vi "Add Component Default Settings.vi"(8 "error in (no error)":errorcluster, 10 "Component":refnum<class "Component.lvclass">, 11 "framework configuration in":T1) -> (0 "error out":errorcluster, 3 "framework configuration out":T1)   [LabVIEW 2017, in "DSF Core.lvlib"]
uses:
  DSF Core.lvlib
  Typedefs/DSF Engine Framework Configuration.ctl
  Typedefs/DSF Settings Info.ctl
  Typedefs/DSF Engine Plugin Configuration.ctl
  Typedefs/DSF Engine Plugin Thread Configuration.ctl
  Typedefs/DSF Engine Transfer Group Configuration.ctl
  Typedefs/DSF Engine Transfer Configuration.ctl
  Typedefs/DSF Engine Channel Configuration.ctl
  Classes/Component/Component.lvclass
  Classes/Configuration/Base/Group/Group Configuration.lvclass
  Classes/Configuration/Configuration.lvclass
  Classes/Component Configuration/Component Configurations.lvclass
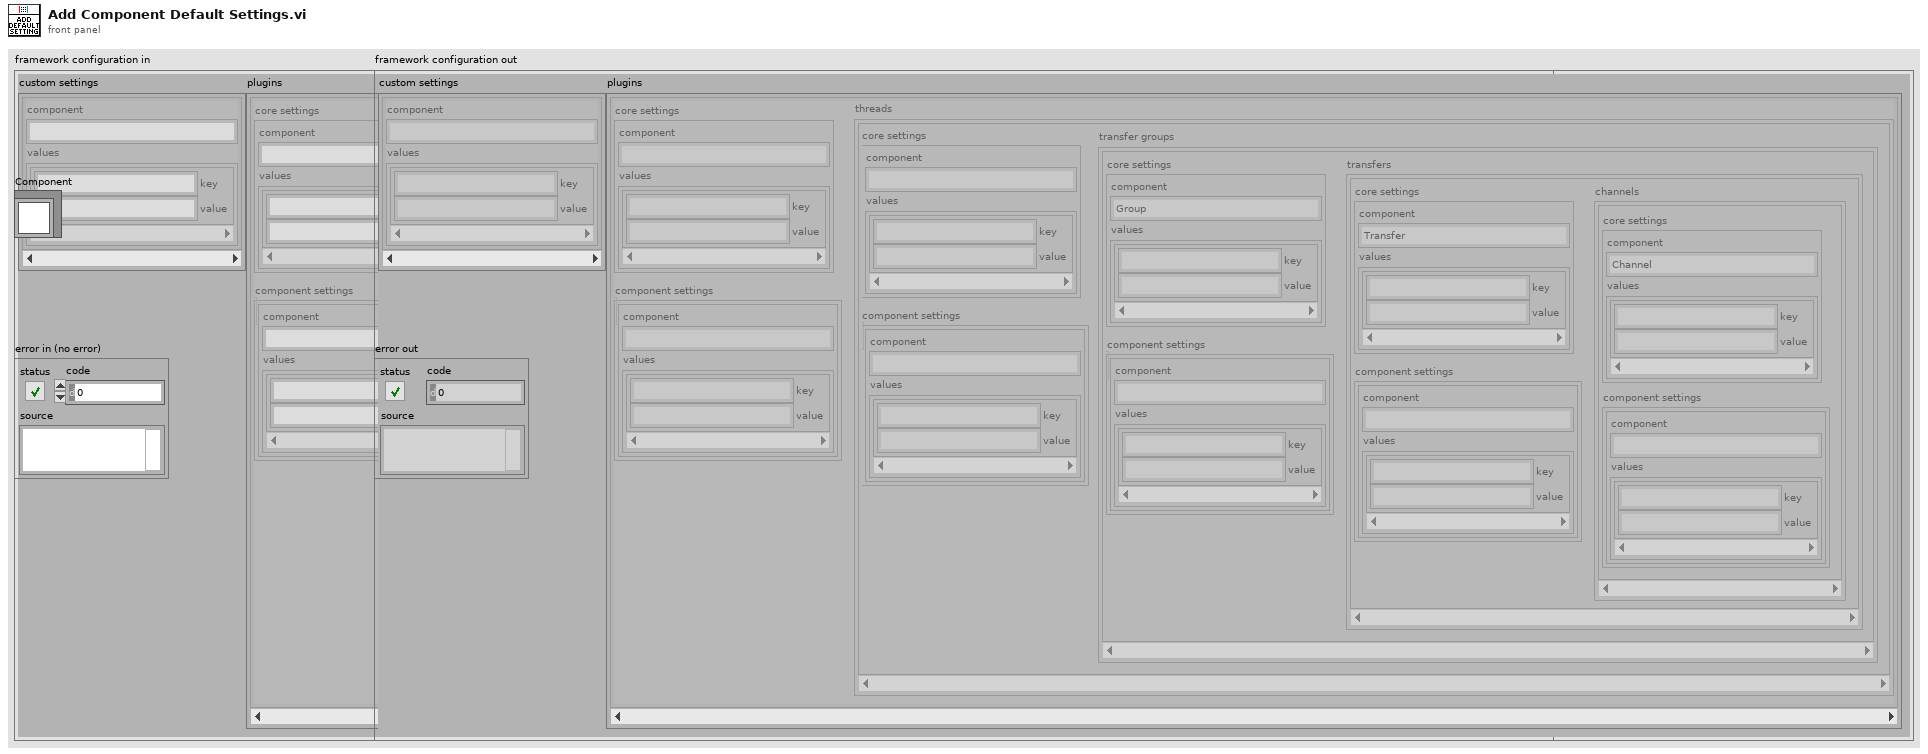
[diagram p1: front panel]
types:
  T1 = typedef "DSF Core.lvlib/DSF Engine Framework Configuration.ctl" = cluster{"custom settings":T2[], "plugins":T3[]}
  T2 = typedef "DSF Core.lvlib/DSF Settings Info.ctl" = cluster{"component":string, "values":cluster{"key":string, "value":string}[]}
  T3 = typedef "DSF Core.lvlib/DSF Engine Plugin Configuration.ctl" = cluster{"core settings":T2, "component settings":T2[], "threads":T4[]}
  T4 = typedef "DSF Core.lvlib/DSF Engine Plugin Thread Configuration.ctl" = cluster{"core settings":T2, "component settings":T2[], "transfer groups":T5[]}
  T5 = typedef "DSF Core.lvlib/DSF Engine Transfer Group Configuration.ctl" = cluster{"core settings":T2, "component settings":T2[], "transfers":T6[]}
  T6 = typedef "DSF Core.lvlib/DSF Engine Transfer Configuration.ctl" = cluster{"core settings":T2, "component settings":T2[], "channels":T7[]}
  T7 = typedef "DSF Core.lvlib/DSF Engine Channel Configuration.ctl" = cluster{"core settings":T2, "component settings":T2[]}
  T8 = typedef "DSF Core.lvlib/Group Configuration.lvclass/Core Group Configuration.ctl" = cluster{"name":string, "direction":T9, "cycle timing":T10, "timeout behavior":T11, "enable conversion":bool}
  T9 = typedef "DSF Core.lvlib/DSF Direction.ctl" = enum8{"Tx", "Rx"}
  T10 = typedef "DSF Core.lvlib/DSF Timing Info.ctl" = cluster{"priority":u64, "decimation":u64, "offset":u64}
  T11 = typedef "DSF Core.lvlib/DSF Timeout Behavior.ctl" = enum8{"Increment Late Count", "Throw Error"}
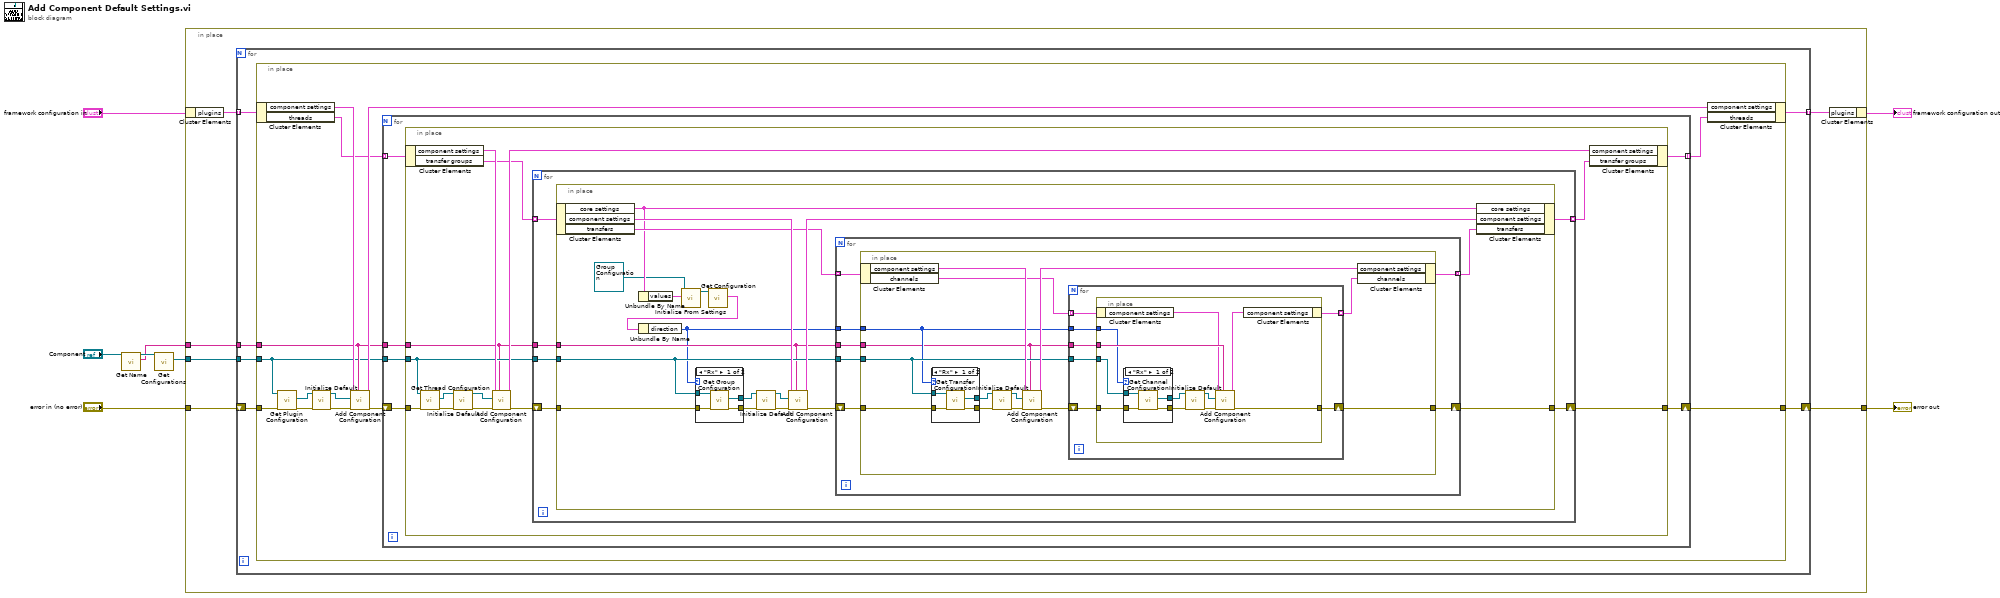
[diagram p0: block diagram]
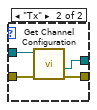
[diagram p2: hidden frame]
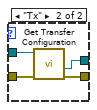
[diagram p3: hidden frame]
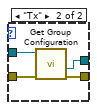
[diagram p4: hidden frame]
diagram:
  n1 = call "Get Name.vi"("Component in"="Component") -> ("name"=w3:string, "Component out"=w5:refnum<class "Component.lvclass">)  [unwired: 9 in]
  n2 = call "Get Configurations.vi"("Component in"=w5) -> ("Configurations"=w4:refnum<class "Component Configurations.lvclass">)  [unwired: 9 in, 1 out]
  n3 = in-place {
    in-place-border: w4 -> [w12]
    in-place-border: w3 -> [w11]
    in-place-border: "error in (no error)" -> [w10]
    in-place-border: [w9] -> w1
    n4 = in-place-cluster #1("framework configuration in") -> ("plugins"=w14:T3[])
    n5 = for {
      tunnel: w14 -> [w19] mode=indexing
      tunnel: [w20] -> w13 mode=indexing
      tunnel: w12 -> [w18]
      tunnel: w11 -> [w17]
      shift-right: [w15] -> w9
      shift-left: w10 -> [w16]
      n6 = in-place {
        in-place-border: w18 -> [w22]
        in-place-border: w17 -> [w24]
        in-place-border: w16 -> [w27]
        in-place-border: [w21] -> w15
        n7 = in-place-cluster #2(w19) -> ("component settings"=w29:T2[], "threads"=w26:T4[])
        n8 = call "Get Plugin Configuration.vi"("error in (no error)"=w27, "Component Configuration in"=w22) -> ("error out"=w32:errorcluster, "Plugin Configuration"=w33:refnum<class "Configuration.lvclass">)  [unwired: 7 in, 1 out]
        n9 = call-dynamic "Initialize Default.vi"("error in (no error)"=w32, "Configuration in"=w33) -> ("error out"=w28:errorcluster, "Configuration out"=w31:refnum<class "Configuration.lvclass">)  [unwired: 8 in]
        n10 = call "Add Component Configuration.vi"("component name"=w24, "error in (no error)"=w28, "Configuration"=w31, "component settings in"=w29) -> ("error out"=w23:errorcluster, "component settings out"=w30:T2[])  [unwired: 5 in, 1 out]
        n11 = for {
          tunnel: w26 -> [w39] mode=indexing
          tunnel: [w38] -> w25 mode=indexing
          tunnel: w24 -> [w37]
          shift-right: [w34] -> w21
          shift-left: w23 -> [w36]
          tunnel: w22 -> [w35]
          n12 = in-place {
            in-place-border: w37 -> [w43]
            in-place-border: w36 -> [w48]
            in-place-border: w35 -> [w44]
            in-place-border: [w41] -> w34
            n13 = in-place-cluster #3(w39) -> ("component settings"=w50:T2[], "transfer groups"=w45:T5[])
            n14 = call "Get Thread Configuration.vi"("error in (no error)"=w48, "Component Configuration in"=w44) -> ("error out"=w47:errorcluster, "Thread Configuration"=w46:refnum<class "Configuration.lvclass">)  [unwired: 7 in, 1 out]
            n15 = call-dynamic "Initialize Default.vi"("error in (no error)"=w47, "Configuration in"=w46) -> ("error out"=w51:errorcluster, "Configuration out"=w52:refnum<class "Configuration.lvclass">)  [unwired: 8 in]
            n16 = call "Add Component Configuration.vi"("component name"=w43, "error in (no error)"=w51, "Configuration"=w52, "component settings in"=w50) -> ("error out"=w42:errorcluster, "component settings out"=w49:T2[])  [unwired: 5 in, 1 out]
            n17 = for {
              tunnel: w45 -> [w58] mode=indexing
              tunnel: w44 -> [w57]
              tunnel: w43 -> [w56]
              shift-right: [w54] -> w41
              shift-left: w42 -> [w55]
              tunnel: [w53] -> w40 mode=indexing
              n18 = in-place {
                in-place-border: w57 -> [w68]
                in-place-border: w56 -> [w67]
                in-place-border: w55 -> [w77]
                in-place-border: [w65] -> w54
                n19 = in-place-cluster #4(w58) -> ("core settings"=w63:T2, "component settings"=w73:T2[], "transfers"=w70:T6[])
                n20 = Unbundle By Name(w63) -> ("values"=w62:cluster{"key":string, "value":string}[])
                n21 = call-dynamic "Initialize From Settings.vi"("settings"=w62, "Core Groups Configuration in"=refnum<class "Group Configuration.lvclass"> refnum) -> ("Core Groups Configuration out"=w61:refnum<class "Group Configuration.lvclass">)  [unwired: 8 in, 1 out]
                n22 = call "Get Configuration.vi"("Core Groups Configuration in"=w61) -> ("configuration"=w60:T8)  [unwired: 8 in, 2 out]
                n23 = Unbundle By Name(w60) -> ("direction"=w66:T9)
                n24 = case shown="\"Rx\"" w66 {
                  tunnel: w68 -> [w135 w139]
                  tunnel: w77 -> [w136 w140]
                  tunnel: [w134 w138] -> w76
                  tunnel: [w133 w137] -> w75
                  frame "Rx" {
                    n25 = call "Get Group Configuration.vi"("error in (no error)"=w136, "Component Configuration in"=w135) -> ("error out"=w134:errorcluster, "Rx Group Configuration"=w133:refnum<class "Configuration.lvclass">)  [unwired: 6 in, 2 out]
                  }
                  frame "Tx" {
                    n26 = call "Get Group Configuration.vi"("error in (no error)"=w140, "Component Configuration in"=w139) -> ("error out"=w138:errorcluster, "Tx Group Configuration"=w137:refnum<class "Configuration.lvclass">)  [unwired: 6 in, 2 out]
                  }
                }
                n27 = call-dynamic "Initialize Default.vi"("error in (no error)"=w76, "Configuration in"=w75) -> ("error out"=w74:errorcluster, "Configuration out"=w71:refnum<class "Configuration.lvclass">)  [unwired: 8 in]
                n28 = call "Add Component Configuration.vi"("component name"=w67, "error in (no error)"=w74, "Configuration"=w71, "component settings in"=w73) -> ("error out"=w69:errorcluster, "component settings out"=w72:T2[])  [unwired: 5 in, 1 out]
                n29 = for {
                  tunnel: w70 -> [w84] mode=indexing
                  tunnel: w66 -> [w83]
                  shift-right: [w79] -> w65
                  shift-left: w69 -> [w82]
                  tunnel: w68 -> [w81]
                  tunnel: w67 -> [w80]
                  tunnel: [w78] -> w64 mode=indexing
                  n30 = in-place {
                    in-place-border: w83 -> [w88]
                    in-place-border: w82 -> [w94]
                    in-place-border: w81 -> [w89]
                    in-place-border: w80 -> [w87]
                    in-place-border: [w86] -> w79
                    n31 = in-place-cluster #5(w84) -> ("component settings"=w93:T2[], "channels"=w91:T7[])
                    n32 = case shown="\"Rx\"" w88 {
                      tunnel: w89 -> [w127 w131]
                      tunnel: w94 -> [w128 w132]
                      tunnel: [w126 w130] -> w98
                      tunnel: [w125 w129] -> w97
                      frame "Rx" {
                        n33 = call "Get Transfer Configuration.vi"("error in (no error)"=w128, "Component Configuration in"=w127) -> ("error out"=w126:errorcluster, "Rx Transfer Configuration"=w125:refnum<class "Configuration.lvclass">)  [unwired: 6 in, 2 out]
                      }
                      frame "Tx" {
                        n34 = call "Get Transfer Configuration.vi"("error in (no error)"=w132, "Component Configuration in"=w131) -> ("error out"=w130:errorcluster, "Tx Transfer Configuration"=w129:refnum<class "Configuration.lvclass">)  [unwired: 6 in, 2 out]
                      }
                    }
                    n35 = call-dynamic "Initialize Default.vi"("error in (no error)"=w98, "Configuration in"=w97) -> ("error out"=w96:errorcluster, "Configuration out"=w95:refnum<class "Configuration.lvclass">)  [unwired: 8 in]
                    n36 = call "Add Component Configuration.vi"("component name"=w87, "error in (no error)"=w96, "Configuration"=w95, "component settings in"=w93) -> ("error out"=w90:errorcluster, "component settings out"=w92:T2[])  [unwired: 5 in, 1 out]
                    n37 = for {
                      tunnel: w91 -> [w105] mode=indexing
                      shift-right: [w103] -> w86
                      shift-left: w90 -> [w104]
                      tunnel: w89 -> [w102]
                      tunnel: w88 -> [w100]
                      tunnel: w87 -> [w101]
                      tunnel: [w99] -> w85 mode=indexing
                      n38 = in-place {
                        in-place-border: w104 -> [w112]
                        in-place-border: [w111] -> w103
                        in-place-border: w102 -> [w110]
                        in-place-border: w101 -> [w109]
                        in-place-border: w100 -> [w108]
                        n39 = in-place-cluster #6(w105) -> ("component settings"=w107:T2[])
                        n40 = case shown="\"Rx\"" w108 {
                          tunnel: w110 -> [w119 w123]
                          tunnel: w112 -> [w120 w124]
                          tunnel: [w117 w122] -> w116
                          tunnel: [w118 w121] -> w115
                          frame "Rx" {
                            n41 = call "Get Channel Configuration.vi"("error in (no error)"=w120, "Component Configuration in"=w119) -> ("error out"=w117:errorcluster, "Rx Channel Configuration"=w118:refnum<class "Configuration.lvclass">)  [unwired: 6 in, 2 out]
                          }
                          frame "Tx" {
                            n42 = call "Get Channel Configuration.vi"("error in (no error)"=w124, "Component Configuration in"=w123) -> ("error out"=w122:errorcluster, "Tx Channel Configuration"=w121:refnum<class "Configuration.lvclass">)  [unwired: 6 in, 2 out]
                          }
                        }
                        n43 = call-dynamic "Initialize Default.vi"("error in (no error)"=w116, "Configuration in"=w115) -> ("error out"=w114:errorcluster, "Configuration out"=w113:refnum<class "Configuration.lvclass">)  [unwired: 8 in]
                        n44 = call "Add Component Configuration.vi"("component name"=w109, "error in (no error)"=w114, "Configuration"=w113, "component settings in"=w107) -> ("error out"=w111:errorcluster, "component settings out"=w106:T2[])  [unwired: 5 in, 1 out]
                        n45 = in-place-cluster #6("component settings"=w106) -> (w99:T7)
                      }
                    }
                    n46 = in-place-cluster #5("component settings"=w92, "channels"=w85) -> (w78:T6)
                  }
                }
                n47 = in-place-cluster #4("core settings"=w63, "component settings"=w72, "transfers"=w64) -> (w53:T5)
              }
            }
            n48 = in-place-cluster #3("component settings"=w49, "transfer groups"=w40) -> (w38:T4)
          }
        }
        n49 = in-place-cluster #2("component settings"=w30, "threads"=w25) -> (w20:T3)
      }
    }
    n50 = in-place-cluster #1("plugins"=w13) -> (→"framework configuration out":T1)
  }
  "error out" <- w1
